vi "ge_LoadRingSupportList.vi"(8 "error in":errorcluster, 11 "RingSupport":T1[](array[typedef])) -> (0 "error out":errorcluster, 3 "List Variant":variant)   [LabVIEW 2018]
uses:
  Custom Ctrls/ge_RingSupport.ctl
  Common/Controls/HeaderNames.ctl
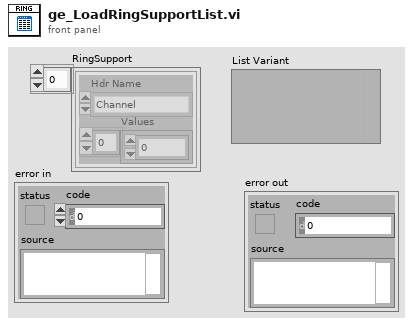
[diagram p1: front panel]
types:
  T1 = typedef "ge_RingSupport.ctl" = cluster{"Hdr Name":T2, "Values":u16[]}
  T2 = typedef "HeaderNames.ctl" = enum16{"Channel", "Device", "Spacer", "Description", "MB", "Range", "Terminal", "Coupling", "Thresh (V)", "Pulse/Rev", "Slope", "Min EU", "Min RPM", "mV/EU", "Iex", "Temp Units", "Type", "CJC Src", "CJC Val", "Ro", "Wire Cfg", "Strain Mode", "Vex", "Bridge Type", "GF", "Gauge Res", "Poisson", "Lead Res", "Init Strain", "GAF", "Scale", "Offset", "Unit (EU)", "dB?", "dB Ref", "Cal Mag", "Cal Units", "Max Temp", "Min Temp", "Max Strain", "Min Strain"}
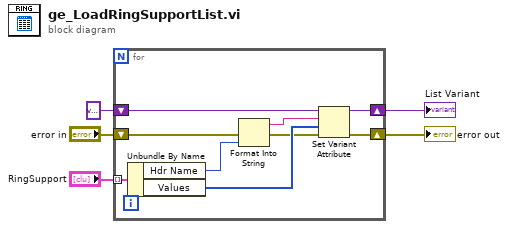
[diagram p0: block diagram]
diagram:
  n1 = for {
    tunnel: "RingSupport" -> [w14] mode=indexing
    shift-right: [w11] -> w5
    shift-left: variant ("variant") -> [w12]
    shift-right: [w7] -> w1
    shift-left: "error in" -> [w6]
    n2 = Unbundle By Name(w14) -> ("Hdr Name"=w10:T2, "Values"=w13:u16[])
    n3 = Format Into String(error in=w6, w10) -> (resulting string=w9:string, error out=w8:errorcluster)  [unwired: 2 in]
    n4 = Set Variant Attribute(Variant=w12, name=w9, value=w13, error in=w8) -> (Variant out=w11:variant, error out=w7:errorcluster)  [unwired: 1 out]
  }
  "List Variant" <- w5
  "error out" <- w1
